vi "Extract White.vi"() -> ()   [LabVIEW 2009]
uses:
  <vilib>/vision/NI_Vision_Development_Module.lvlib
panel:
  out "Result":T1(plugin-control)
  out "LH":sgl[][](array[numeric]) format="%.2f"
  out "test":T1(plugin-control)
  in  "Size & Tolerance":T2={"X Size"=3, "Y Size"=3, "% Tolerance"=40}
  in  "stop 2":bool
  out "BlueEqLow":T1(plugin-control)
  out "BlueEq":T3(graph)
  out "BlueEq":T1(plugin-control)
  in  "stop":bool
  out "BlueEqLowThres":T1(plugin-control)
  out "Lum":T1(plugin-control)
  out "Sat":T1(plugin-control)
  out "Hue":T1(plugin-control)
  out "Blue":T1(plugin-control)
  out "Green":T1(plugin-control)
  out "Red":T1(plugin-control)
  in  "Manual":cluster{"Min":i32, "Max":i32}(slide)={"Min"=0, "Max"=150} caption="Threshold Range" scale=0.0..255.0
  out "Hue":T3(graph)
  out "Sat":T3(graph)
  out "Luma":T3(graph)
  out "Blue":T3(graph)
  out "Green":T3(graph)
  out "Red":T3(graph)
  out "Original":T1(plugin-control)
  in  "File Path":path
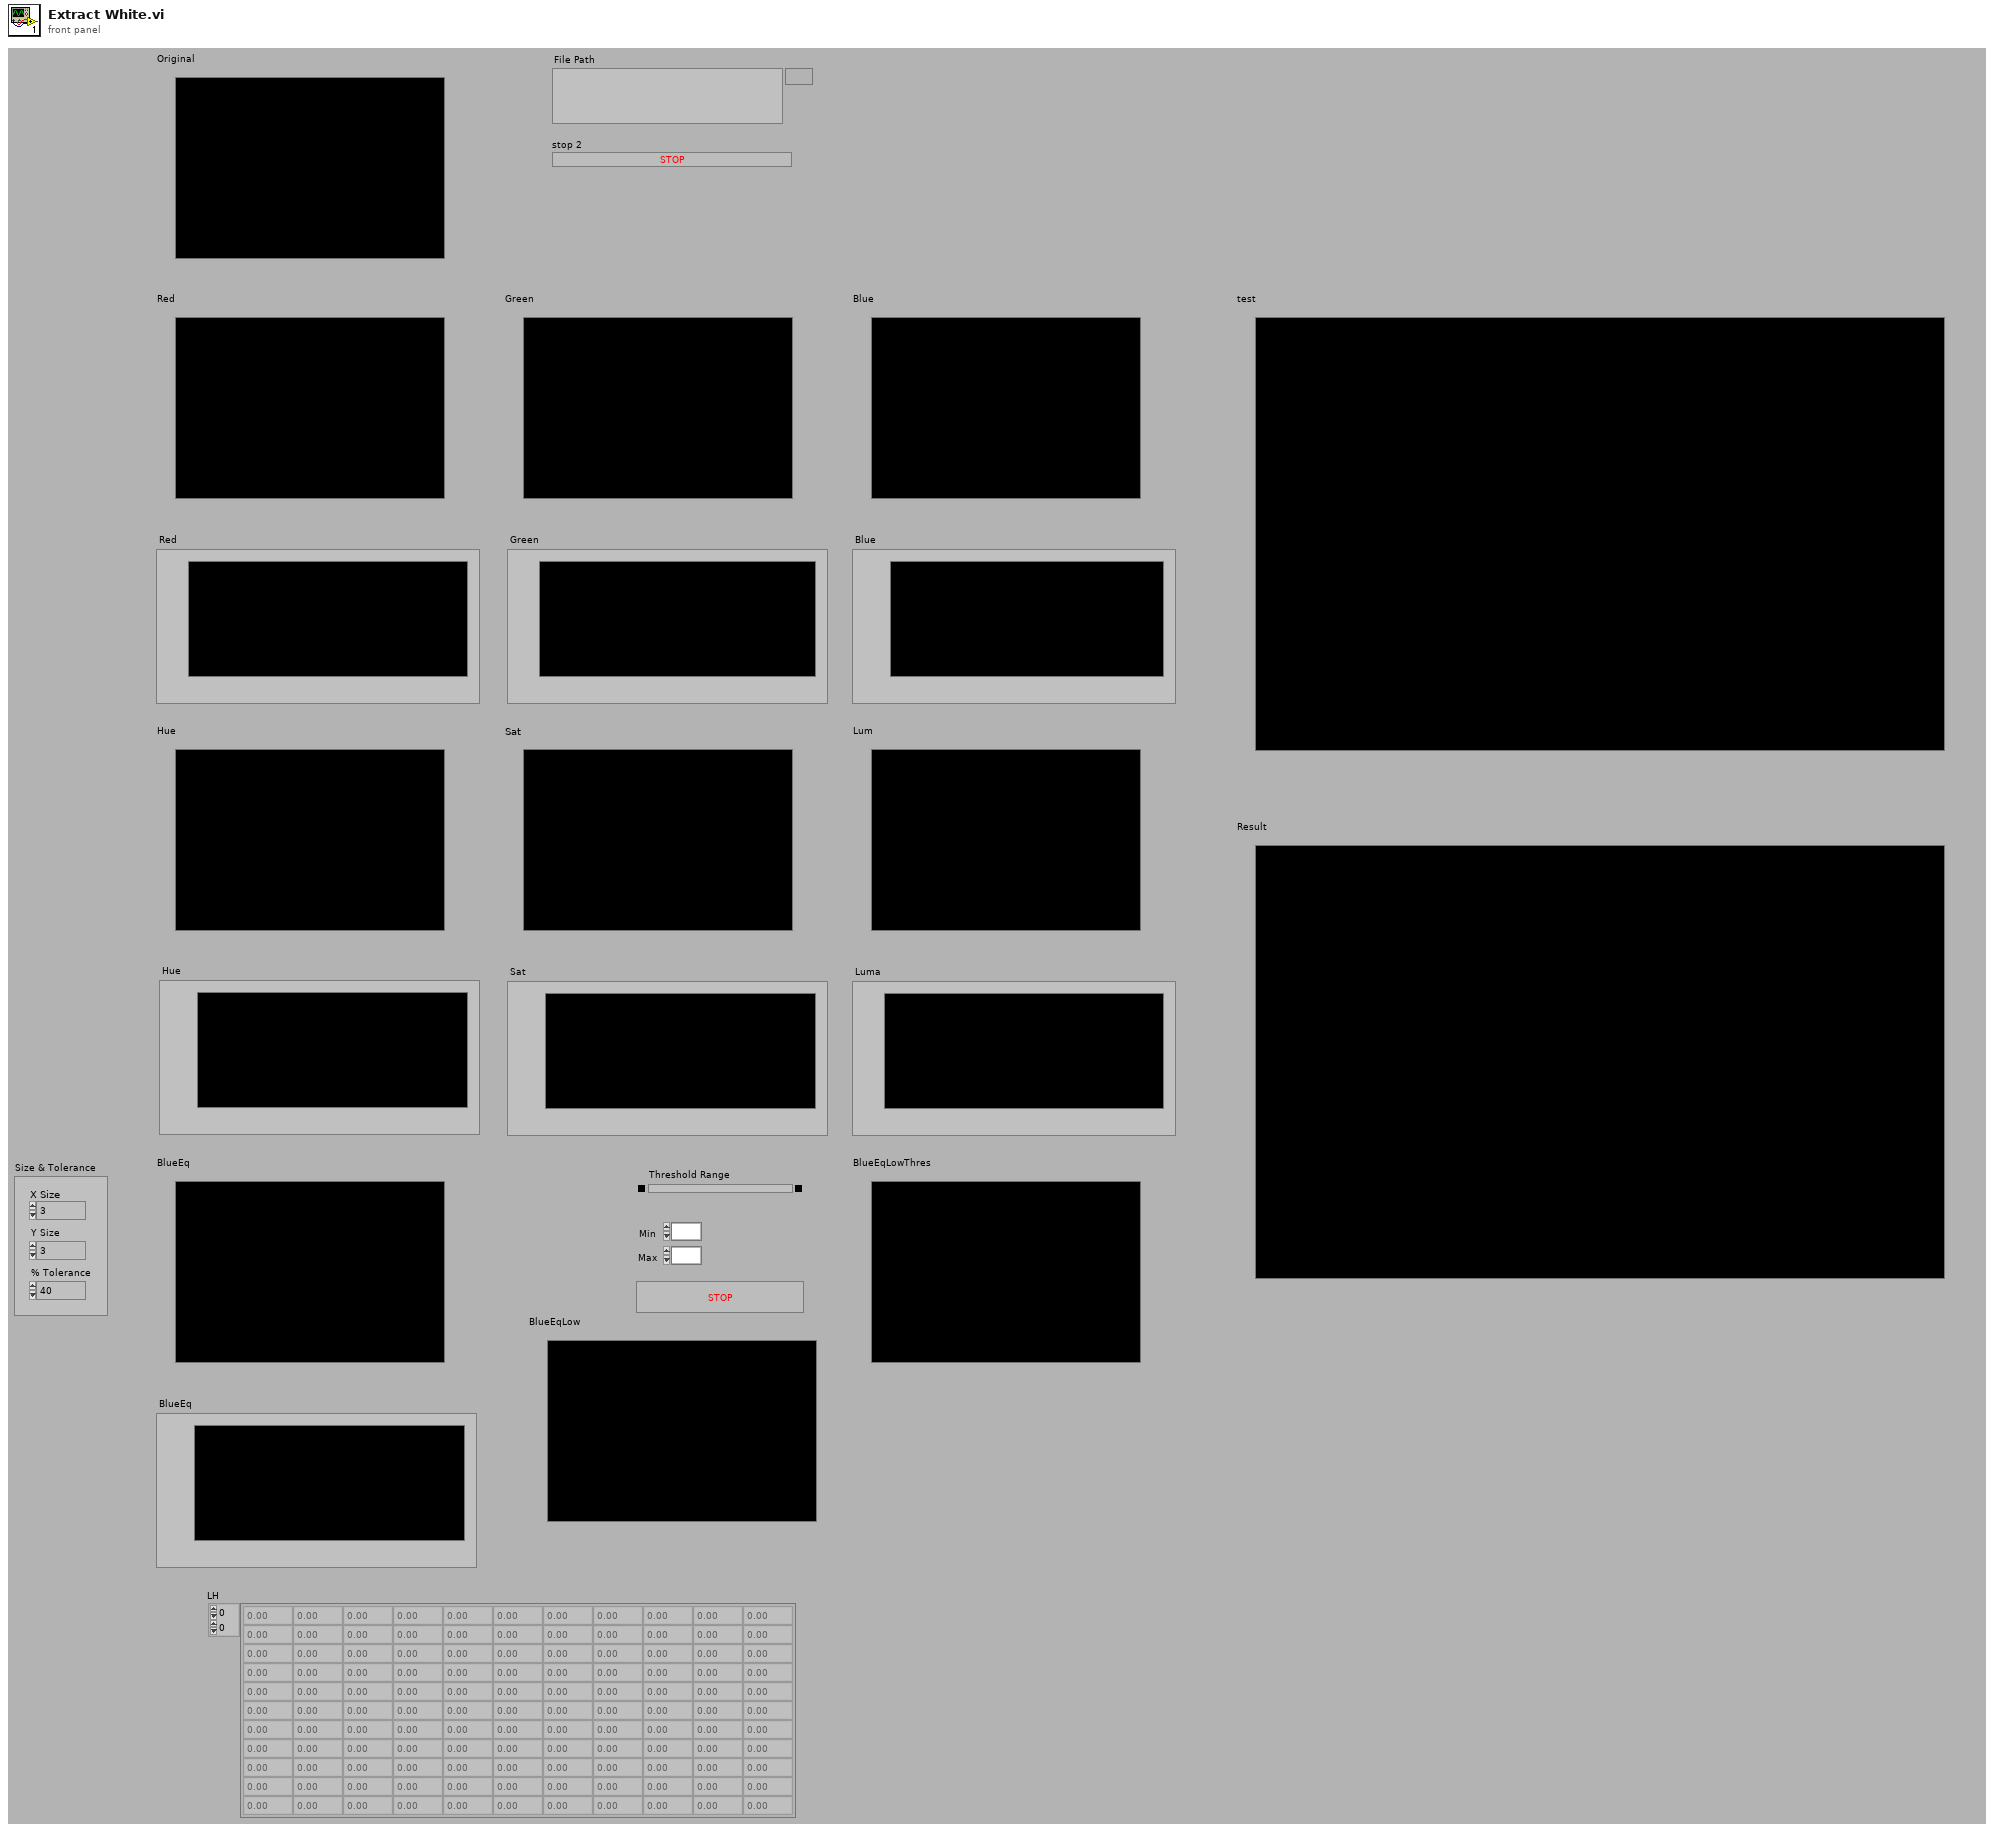
[diagram p1: front panel]
types:
  T1 = typedef "IMAQ Image.ctl" = refnum<image>
  T2 = cluster{"X Size":i32, "Y Size":i32, "% Tolerance":i32}
  T3 = cluster{"Starting Value":sgl, "Incremental Value":sgl, "Histogram":u32[]}
  T4 = typedef "Image Type" = u32
  T5 = cluster{"Type":i32, "Wavelet Bands To Use":i32[], "Min. Energy Level":sgl}
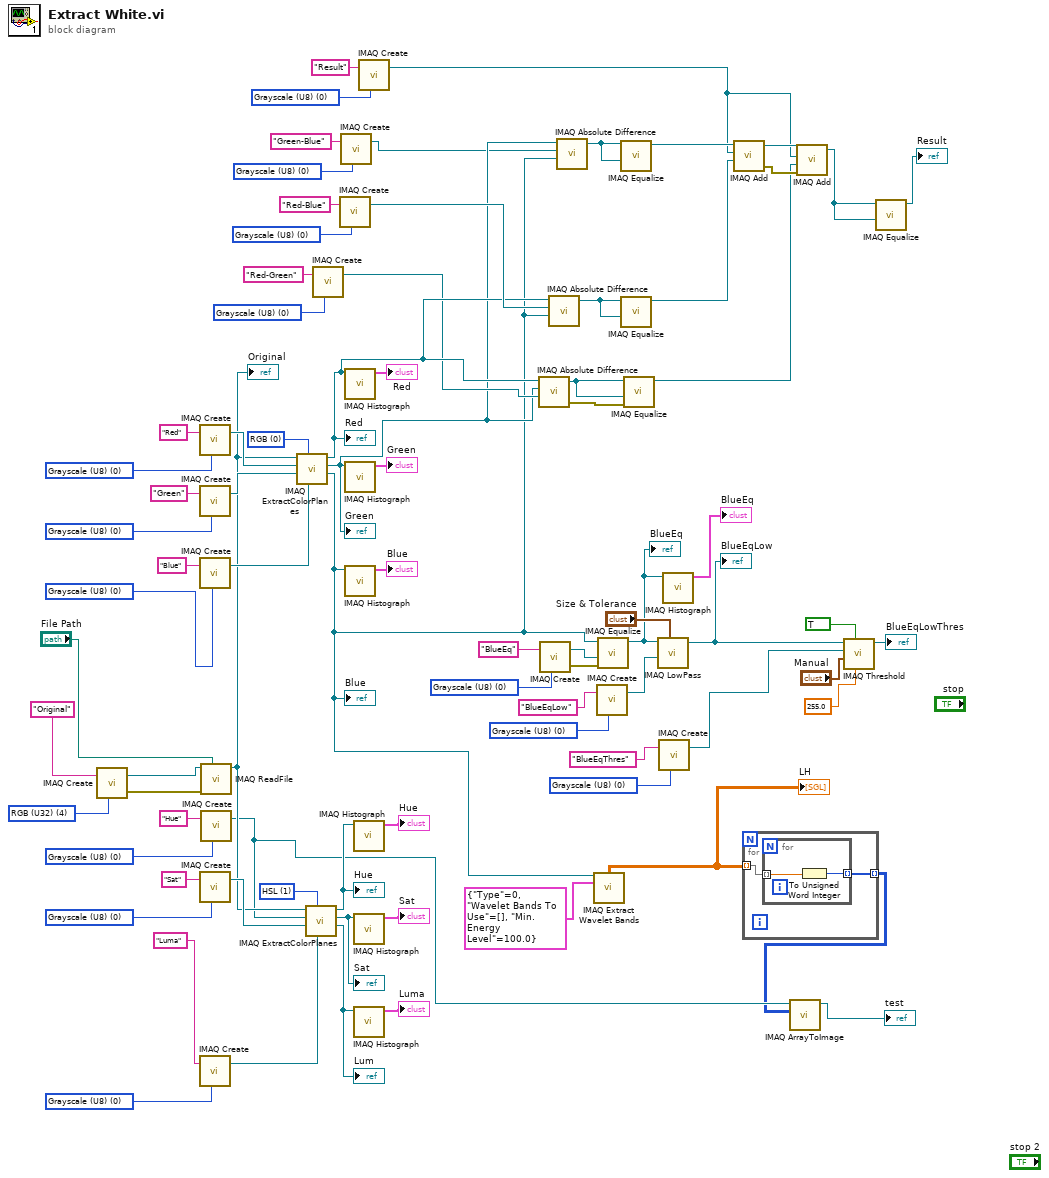
[diagram p0: block diagram]
diagram:
  w8 = T4 0 items=["Grayscale (U8)", "Grayscale (I16)", "Grayscale (SGL)", "Complex (CSG)", "RGB (U32)", "HSL (U32)", "RGB (U64)", "Grayscale (U16)"] ("Image Type")
  w22 = T4 0 items=["Grayscale (U8)", "Grayscale (I16)", "Grayscale (SGL)", "Complex (CSG)", "RGB (U32)", "HSL (U32)", "RGB (U64)", "Grayscale (U16)"] ("Image Type")
  w23 = T4 0 items=["Grayscale (U8)", "Grayscale (I16)", "Grayscale (SGL)", "Complex (CSG)", "RGB (U32)", "HSL (U32)", "RGB (U64)", "Grayscale (U16)"] ("Image Type")
  w26 = T4 0 items=["Grayscale (U8)", "Grayscale (I16)", "Grayscale (SGL)", "Complex (CSG)", "RGB (U32)", "HSL (U32)", "RGB (U64)", "Grayscale (U16)"] ("Image Type")
  w45 = T4 0 items=["Grayscale (U8)", "Grayscale (I16)", "Grayscale (SGL)", "Complex (CSG)", "RGB (U32)", "HSL (U32)", "RGB (U64)", "Grayscale (U16)"] ("Image Type")
  w49 = T4 0 items=["Grayscale (U8)", "Grayscale (I16)", "Grayscale (SGL)", "Complex (CSG)", "RGB (U32)", "HSL (U32)", "RGB (U64)", "Grayscale (U16)"] ("Image Type")
  w55 = T4 0 items=["Grayscale (U8)", "Grayscale (I16)", "Grayscale (SGL)", "Complex (CSG)", "RGB (U32)", "HSL (U32)", "RGB (U64)", "Grayscale (U16)"] ("Image Type")
  w70 = u16 1 items=["RGB", "HSL", "HSV", "HSI"] ("Color Mode")
  w66 = T4 0 items=["Grayscale (U8)", "Grayscale (I16)", "Grayscale (SGL)", "Complex (CSG)", "RGB (U32)", "HSL (U32)", "RGB (U64)", "Grayscale (U16)"] ("Image Type")
  w65 = T4 0 items=["Grayscale (U8)", "Grayscale (I16)", "Grayscale (SGL)", "Complex (CSG)", "RGB (U32)", "HSL (U32)", "RGB (U64)", "Grayscale (U16)"] ("Image Type")
  w62 = T4 0 items=["Grayscale (U8)", "Grayscale (I16)", "Grayscale (SGL)", "Complex (CSG)", "RGB (U32)", "HSL (U32)", "RGB (U64)", "Grayscale (U16)"] ("Image Type")
  w71 = u16 0 items=["RGB", "HSL", "HSV", "HSI"] ("Color Mode")
  w76 = T4 0 items=["Grayscale (U8)", "Grayscale (I16)", "Grayscale (SGL)", "Complex (CSG)", "RGB (U32)", "HSL (U32)", "RGB (U64)", "Grayscale (U16)"] ("Image Type")
  w77 = T4 0 items=["Grayscale (U8)", "Grayscale (I16)", "Grayscale (SGL)", "Complex (CSG)", "RGB (U32)", "HSL (U32)", "RGB (U64)", "Grayscale (U16)"] ("Image Type")
  w80 = T4 0 items=["Grayscale (U8)", "Grayscale (I16)", "Grayscale (SGL)", "Complex (CSG)", "RGB (U32)", "HSL (U32)", "RGB (U64)", "Grayscale (U16)"] ("Image Type")
  w81 = T4 4 items=["Grayscale (U8)", "Grayscale (I16)", "Grayscale (SGL)", "Complex (CSG)", "RGB (U32)", "HSL (U32)", "RGB (U64)", "Grayscale (U16)"] ("Image Type")
  n1 = call "IMAQ Create"("Image Name"="Original", "Image Type"=w81) -> ("New Image"=w36:T1, "error out"=w83:errorcluster)  [unwired: 3 in]
  n2 = call "IMAQ Create"("Image Name"="Red", "Image Type"=w80) -> ("New Image"=w74:T1)  [unwired: 3 in, 1 out]
  n3 = call "IMAQ Create"("Image Name"="Green", "Image Type"=w77) -> ("New Image"=w73:T1)  [unwired: 3 in, 1 out]
  n4 = call "IMAQ Create"("Image Name"="Blue", "Image Type"=w76) -> ("New Image"=w72:T1)  [unwired: 3 in, 1 out]
  n5 = call "IMAQ Create"("Image Name"="Sat", "Image Type"=w65) -> ("New Image"=w68:T1)  [unwired: 3 in, 1 out]
  n6 = call "IMAQ Create"("Image Name"="Luma", "Image Type"=w66) -> ("New Image"=w69:T1)  [unwired: 3 in, 1 out]
  n7 = call "IMAQ ReadFile"("File Path"="File Path", "error in (no error)"=w83, "Image"=w36) -> ("Image Out"=w61:T1)  [unwired: 4 in, 4 out]
  "Original" <- w61
  n8 = call "IMAQ Create"("Image Name"="Hue", "Image Type"=w62) -> ("New Image"=w34:T1)  [unwired: 3 in, 1 out]
  n9 = call "IMAQ ExtractColorPlanes"("Blue or Luma or Val or Inten Plane"=w72, "Color Mode"=w71, "Green or Sat Plane"=w73, "Red or Hue Plane"=w74, "Image Src"=w61) -> ("Blue or Luma or Val or Inten Plane out"=w14:T1, "Green or Sat Plane out"=w15:T1, "Red or Hue Plane out"=w17:T1)  [unwired: 3 in, 1 out]
  "Red" <- w17
  "Green" <- w15
  "Blue" <- w14
  n10 = call "IMAQ ExtractColorPlanes"("Blue or Luma or Val or Inten Plane"=w69, "Color Mode"=w70, "Green or Sat Plane"=w68, "Red or Hue Plane"=w34, "Image Src"=w61) -> ("Blue or Luma or Val or Inten Plane out"=w52:T1, "Green or Sat Plane out"=w51:T1, "Red or Hue Plane out"=w37:T1)  [unwired: 3 in, 1 out]
  "Hue" <- w37
  "Sat" <- w51
  "Lum" <- w52
  n11 = call "IMAQ Create"("Image Name"="Red-Green", "Image Type"=w26) -> ("New Image"=w16:T1)  [unwired: 3 in, 1 out]
  n12 = call "IMAQ Create"("Image Name"="Red-Blue", "Image Type"=w23) -> ("New Image"=w20:T1)  [unwired: 3 in, 1 out]
  n13 = call "IMAQ Create"("Image Name"="Green-Blue", "Image Type"=w22) -> ("New Image"=w13:T1)  [unwired: 3 in, 1 out]
  n14 = call "IMAQ Histograph"("Image"=w17) -> ("Histogram Graph"=→"Red":T3)  [unwired: 4 in, 6 out]
  n15 = call "IMAQ Histograph"("Image"=w15) -> ("Histogram Graph"=→"Green":T3)  [unwired: 4 in, 6 out]
  n16 = call "IMAQ Histograph"("Image"=w14) -> ("Histogram Graph"=→"Blue":T3)  [unwired: 4 in, 6 out]
  n17 = call "IMAQ Histograph"("Image"=w37) -> ("Histogram Graph"=→"Hue":T3)  [unwired: 4 in, 6 out]
  n18 = call "IMAQ Histograph"("Image"=w51) -> ("Histogram Graph"=→"Sat":T3)  [unwired: 4 in, 6 out]
  n19 = call "IMAQ Histograph"("Image"=w52) -> ("Histogram Graph"=→"Luma":T3)  [unwired: 4 in, 6 out]
  n20 = call "IMAQ Create"("Image Name"="Result", "Image Type"=w8) -> ("New Image"=w4:T1)  [unwired: 3 in, 1 out]
  n21 = call "IMAQ Absolute Difference"("Image Src A"=w17, "Image Dst"=w15, "Image Src B"=w16) -> ("Image Dst Out"=w19:T1, "error out"=w18:errorcluster)  [unwired: 4 in]
  n22 = call "IMAQ Create"("Image Name"="BlueEq", "Image Type"=w49) -> ("New Image"=w48:T1, "error out"=w47:errorcluster)  [unwired: 3 in]
  n23 = call "IMAQ Absolute Difference"("Image Src A"=w17, "Image Dst"=w20, "Image Src B"=w14) -> ("Image Dst Out"=w12:T1)  [unwired: 4 in, 1 out]
  n24 = call "IMAQ Absolute Difference"("Image Src A"=w15, "Image Dst"=w13, "Image Src B"=w14) -> ("Image Dst Out"=w11:T1)  [unwired: 4 in, 1 out]
  n25 = call "IMAQ Extract Wavelet Bands"("Image"=w14, "Wavelet Options"=T5 {"Type"=0, "Wavelet Bands To Use"=[], "Min. Energy Level"=100.0}) -> ("LL"=w28:sgl[][])  [unwired: 5 in, 8 out]
  "LH" <- w28
  n26 = call "IMAQ Create"("Image Name"="BlueEqLow", "Image Type"=w45) -> ("New Image"=w44:T1)  [unwired: 3 in, 1 out]
  n27 = call "IMAQ Equalize"("error in (no error)"=w47, "Image Dst"=w48, "Image Src"=w14) -> ("Image Dst Out"=w40:T1)  [unwired: 7 in, 1 out]
  "BlueEq" <- w40
  n28 = call "IMAQ Equalize"("Image Dst"=w11, "Image Src"=w11) -> ("Image Dst Out"=w10:T1)  [unwired: 8 in, 1 out]
  n29 = call "IMAQ Equalize"("Image Dst"=w12, "Image Src"=w12) -> ("Image Dst Out"=w7:T1)  [unwired: 8 in, 1 out]
  n30 = call "IMAQ Equalize"("error in (no error)"=w18, "Image Dst"=w19, "Image Src"=w19) -> ("Image Dst Out"=w3:T1)  [unwired: 7 in, 1 out]
  n31 = call "IMAQ LowPass"("Image Src"=w40, "Size & Tolerance"="Size & Tolerance", "Image Dst"=w44) -> ("Image Dst Out"=w39:T1)  [unwired: 4 in, 1 out]
  "BlueEqLow" <- w39
  n32 = call "IMAQ Create"("Image Name"="BlueEqThres", "Image Type"=w55) -> ("New Image"=w53:T1)  [unwired: 3 in, 1 out]
  n33 = call "IMAQ Histograph"("Image"=w40) -> ("Histogram Graph"=→"BlueEq":T3)  [unwired: 4 in, 6 out]
  n34 = call "IMAQ Add"("Image Src A"=w10, "Image Dst"=w4, "Image Src B"=w7) -> ("Image Dst Out"=w6:T1, "error out"=w5:errorcluster)  [unwired: 4 in]
  n35 = for {
    tunnel: w28 -> [w85] mode=indexing
    tunnel: [w84] -> w33 mode=indexing
    n36 = for {
      tunnel: w85 -> [w86] mode=indexing
      tunnel: [w87] -> w84 mode=indexing
      n37 = To Unsigned Word Integer(number=w86) -> (unsigned 16bit integer=w87:u16)
    }
  }
  n38 = call "IMAQ ArrayToImage"("Image Pixels (U8)"=w33, "Image"=w34) -> ("Image Out"=→"test":T1)  [unwired: 8 in, 1 out]
  n39 = call "IMAQ Add"("Image Src A"=w6, "Image Dst"=w4, "Image Src B"=w3, "error in (no error)"=w5) -> ("Image Dst Out"=w2:T1)  [unwired: 3 in, 1 out]
  n40 = call "IMAQ Threshold"("Replace Value"=sgl 255.0, "Keep/Replace Value (Replace)"=TRUE, "Range"="Manual", "Image Dst"=w53, "Image Src"=w39) -> ("Image Dst Out"=→"BlueEqLowThres":T1)  [unwired: 5 in, 1 out]
  n41 = call "IMAQ Equalize"("Image Dst"=w2, "Image Src"=w2) -> ("Image Dst Out"=→"Result":T1)  [unwired: 8 in, 1 out]
